vi "CRYharmonic curves clipf.vi"(9 "Fs":dbl format="%.2f", 10 "Harmonics":dbl[](array[numeric]) format="%.2f", 11 "Freq resp curves":cluster{cluster{"x":dbl, "y":dbl, "z":dbl}[]}[](array[cluster]) {"?"."z" format="%.2f"; "?"."y" format="%.2f"; "?"."x" format="%.2f"}) -> (3 "Freq resp curves clipped":cluster{cluster{"x":dbl, "y":dbl, "z":dbl}[]}[](array[cluster]) {"?"."z" format="%.2f"; "?"."y" format="%.2f"; "?"."x" format="%.2f"})   [LabVIEW 2013]
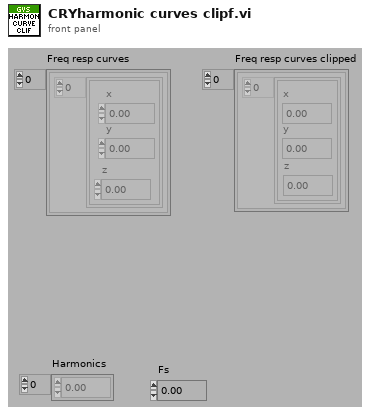
[diagram p1: front panel]
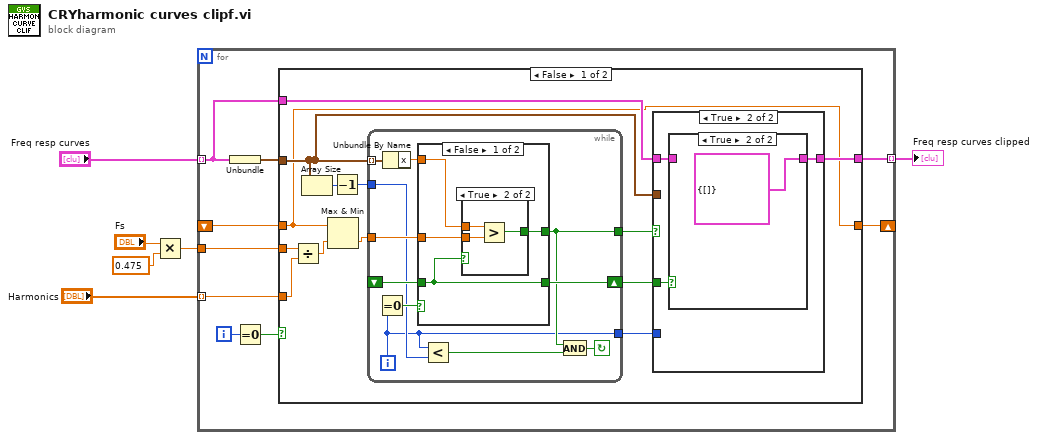
[diagram p0: block diagram]
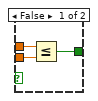
[diagram p2: hidden frame]
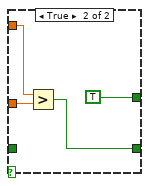
[diagram p3: hidden frame]
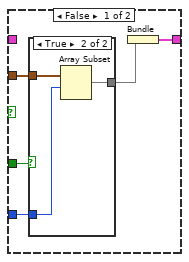
[diagram p4: hidden frame]
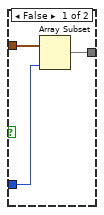
[diagram p5: hidden frame]
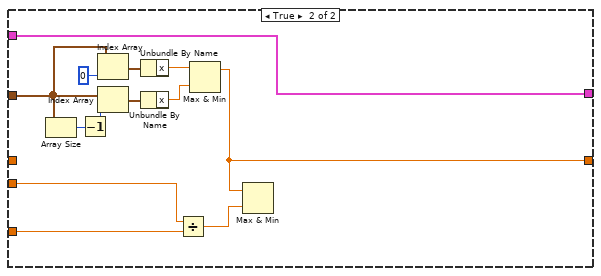
[diagram p7: hidden frame]
diagram:
  n1 = Multiply(x="Fs", y=0.475) -> (x*y=w3:dbl)
  n2 = for {
    tunnel: "Freq resp curves" -> [w8] mode=indexing
    tunnel: w3 -> [w13]
    shift-right: [w12] -> _
    shift-left: _ -> [w11]
    tunnel: "Harmonics" -> [w9] mode=indexing
    tunnel: [w7] -> w2 mode=indexing
    i -> [w10]
    n3 = Unbundle(w8) -> (w14:cluster{"x":dbl, "y":dbl, "z":dbl}[])
    n4 = Equal To 0?(x=w10) -> (x = 0?=w15:bool)
    n5 = case shown="False" w15 {
      tunnel: w14 -> [w20 w75]
      tunnel: w13 -> [w19 w73]
      tunnel: [w18 w70] -> w12
      tunnel: w11 -> [w18 _]
      tunnel: w9 -> [w28 w72]
      tunnel: w8 -> [w23 w74]
      tunnel: [w24 w74] -> w7
      frame False {
        n6 = Divide(x=w19, y=w28) -> (x/y=w16:dbl)
        n7 = Array Size(array=w20) -> (size(s)=w27:i32)
        n8 = Max & Min(x=w18, y=w16) -> (min(x,y)=w17:dbl)  [unwired: 1 out]
        n9 = Decrement(x=w27) -> (x-1=w26:i32)
        n10 = while {
          tunnel: [w29] -> w22
          tunnel: [w30] -> w25
          shift-left: _ -> [w36]
          shift-right: [w37] -> w21
          tunnel: w26 -> [w33]
          tunnel: w17 -> [w38]
          tunnel: w20 -> [w34] mode=indexing
          i -> [w29]
          stop <- w31 continue-if-true
          n11 = Equal To 0?(x=w29) -> (x = 0?=w39:bool)
          n12 = Unbundle By Name(w34) -> ("x"=w35:dbl)
          n13 = case shown="False" w39 {
            tunnel: w38 -> [w42 w53]
            tunnel: [w43 w52] -> w37
            tunnel: w36 -> [w43 _]
            tunnel: w35 -> [w41 w51]
            tunnel: [w40 TRUE] -> w30
            frame False {
              n14 = case shown="True" w43 {
                tunnel: w42 -> [w45 w49]
                tunnel: w41 -> [w46 w48]
                tunnel: [w44 w47] -> w40
                frame False {
                  n15 = Less Or Equal?(x=w46, y=w45) -> (x <= y?=w44:bool)
                }
                frame True {
                  n16 = Greater?(x=w48, y=w49) -> (0:w47:bool)
                }
              }
            }
            frame True {
              n17 = Greater?(x=w51, y=w53) -> (0:w52:bool)
            }
          }
          n18 = Less?(x=w29, y=w33) -> (x < y?=w32:bool)
          n19 = And(x=w30, y=w32) -> (x .and. y?=w31:bool)
        }
        n20 = case shown="True" w25 {
          tunnel: w23 -> [_ w66]
          tunnel: [w55 w65] -> w24
          tunnel: w22 -> [w56 _]
          tunnel: w21 -> [w58 w67]
          tunnel: w20 -> [w57 _]
          frame False {
            n21 = case shown="True" w58 {
              tunnel: w57 -> [w60 w64]
              tunnel: w56 -> [w61 w63]
              tunnel: [w59 w62] -> w54
              frame False {
                n22 = Array Subset(array=w60, length=w61) -> (w59:cluster{"x":dbl, "y":dbl, "z":dbl}[])  [unwired: 1 in]
              }
              frame True {
                n23 = Array Subset(array=w64, index=w63) -> (w62:cluster{"x":dbl, "y":dbl, "z":dbl}[])  [unwired: 1 in]
              }
            }
            n24 = Bundle(w54) -> (w55:cluster{cluster{"x":dbl, "y":dbl, "z":dbl}[]})  [unwired: 1 in]
          }
          frame True {
            n25 = case shown="True" w67 {
              tunnel: w66 -> [w68 _]
              tunnel: [w68 cluster{cluster{"x":dbl, "y":dbl, "z 2":dbl}[]} {[]}] -> w65
              frame False {
              }
              frame True {
              }
            }
          }
        }
      }
      frame True {
        n26 = Array Size(array=w75) -> (size(s)=w82:i32)
        n27 = Decrement(x=w82) -> (x-1=w81:i32)
        n28 = Index Array(array=w75, index=0 ("Index")) -> (element=w78:cluster{"x":dbl, "y":dbl, "z":dbl})
        n29 = Index Array(array=w75, index=w81) -> (element=w80:cluster{"x":dbl, "y":dbl, "z":dbl})
        n30 = Unbundle By Name(w78) -> ("x"=w77:dbl)
        n31 = Unbundle By Name(w80) -> ("x"=w76:dbl)
        n32 = Divide(x=w73, y=w72) -> (x/y=w71:dbl)
        n33 = Max & Min(x=w77, y=w76) -> (max(x,y)=w70:dbl)  [unwired: 1 out]
        n34 = Max & Min(x=w70, y=w71) -> ()  [unwired: 2 out]
      }
    }
  }
  "Freq resp curves clipped" <- w2
